vi "Vision Processing.vi"(4 "error in (no error)":errorcluster, 5 "Camera Type":enum16{"206", "1011", "1013"}(ring)=enum."1011") -> ()   [LabVIEW 2012]
uses:
  Robot Global Data.vi
  <vilib>/vision/NI_Vision_Development_Module.lvlib
panel:
  out "Out Cirlcle Info":cluster{dbl, dbl}
  out "Circle Info":cluster{dbl, dbl, dbl}[](array[cluster])
  in  "Range":cluster{"Lower value":sgl, "Upper value":sgl}={"Lower value"=151.52174, "Upper value"=255.0} {"Lower value" scale=0.0..255.0; "Upper value" scale=0.0..255.0}
  out "Out Target Info":cluster{"X":dbl, "Y":dbl, "Distance (ft)":dbl}
  in  "Enable Vision":bool=TRUE
  in  "View":bool
  out "Target Info":T1(array[cluster])
  in  "Area Size Limit %":dbl=0.5
  in  "Particle Count Limit":i32=8
  in  "Score Limits":T2={"Rect Coverage"=60.0, "X Edge Strength"=40.0, "Y Edge Strength"=60.0, "Center"=33.0, "Outer"=50.0}
  in  "View":bool
  out "Processed Image":T3(plugin-control)
  out "Original Image":T3(plugin-control)
  # "Instructions:\nProcessing the reflective tape that is illuminated by a ring light can be based\non color or light intensity.\nParticles within the image are scored by rectangle coverage, aspect ratio, and\nfor being hollow with a bold edge. A particle is considered a target if all scores\nare above the score limits. Particles can be annotated -- surrounded by\na rectangle and scores drawn to the left .\nTo control the number of particles being scored, use the count limit and the size\nlimit."
  # "To debug, Enable using the View button.\nFor color processing, you can click in the image to select the color for processing."
  # "Enable by clicking the View button.\nGreen scores are above the limit, orange are below. Inner/outer rect\nindicates all passed."
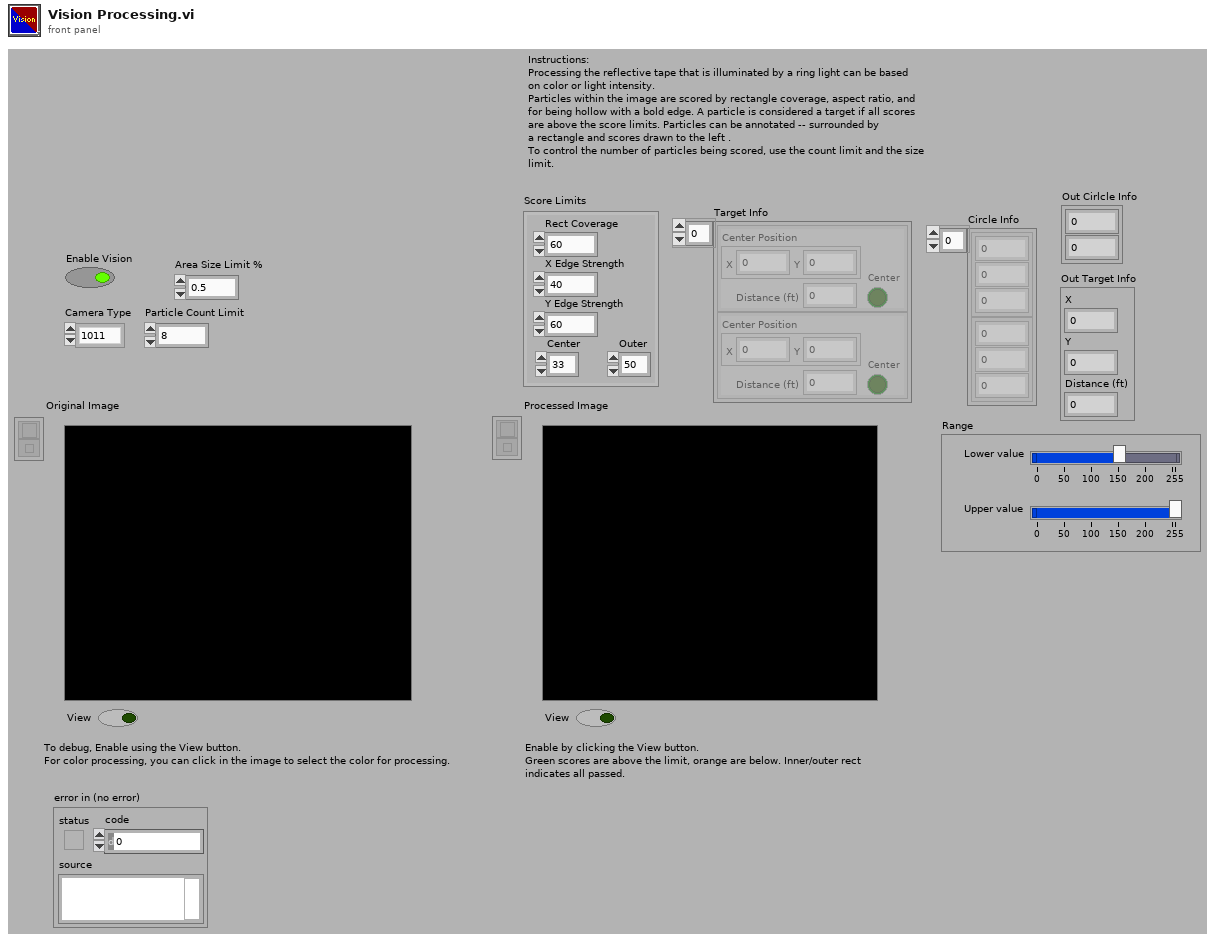
[diagram p1: front panel]
types:
  T1 = cluster{"Center Position":cluster{"X":dbl, "Y":dbl}, "Distance (ft)":dbl, "Center":bool}[]
  T2 = cluster{"Rect Coverage":dbl, "X Edge Strength":dbl, "Y Edge Strength":dbl, "Center":dbl, "Outer":dbl}
  T3 = typedef "IMAQ Image.ctl" = refnum<image>
  T4 = typedef "Image Type" = u32
  T5 = typedef "WPI_CameraDevRef.ctl" = cluster{"Camera Address":string, "CameraStatus":errorcluster, "Acquire Image Notifier":refnum<notifier>}
  T6 = cluster{"Position":cluster{"X":dbl, "Y":dbl}, "Distance (ft)":dbl, "Center":bool}[]
  T7 = typedef "WPI_CameraImageSize.ctl" = enum16{"640x480", "320x240", "160x120"}
  T8 = cluster{cluster{"Left":dbl, "Top":dbl, "Right":dbl, "Bottom":dbl}, "Scores":dbl[], cluster{"Long":dbl, "Short":dbl}}[]
  T9 = cluster{"Target Center (-1 to 1)":cluster{"X":dbl, "Y":dbl}, "Distance (ft)":dbl, "Center Target":bool}
  T10 = cluster{"Target Center (-1 to 1)":cluster{"X":dbl, "Y":dbl}, "Distance (ft)":dbl, "Center Target":bool}[]
  T11 = cluster{"Left":dbl, "Top":dbl, "Right":dbl, "Bottom":dbl}
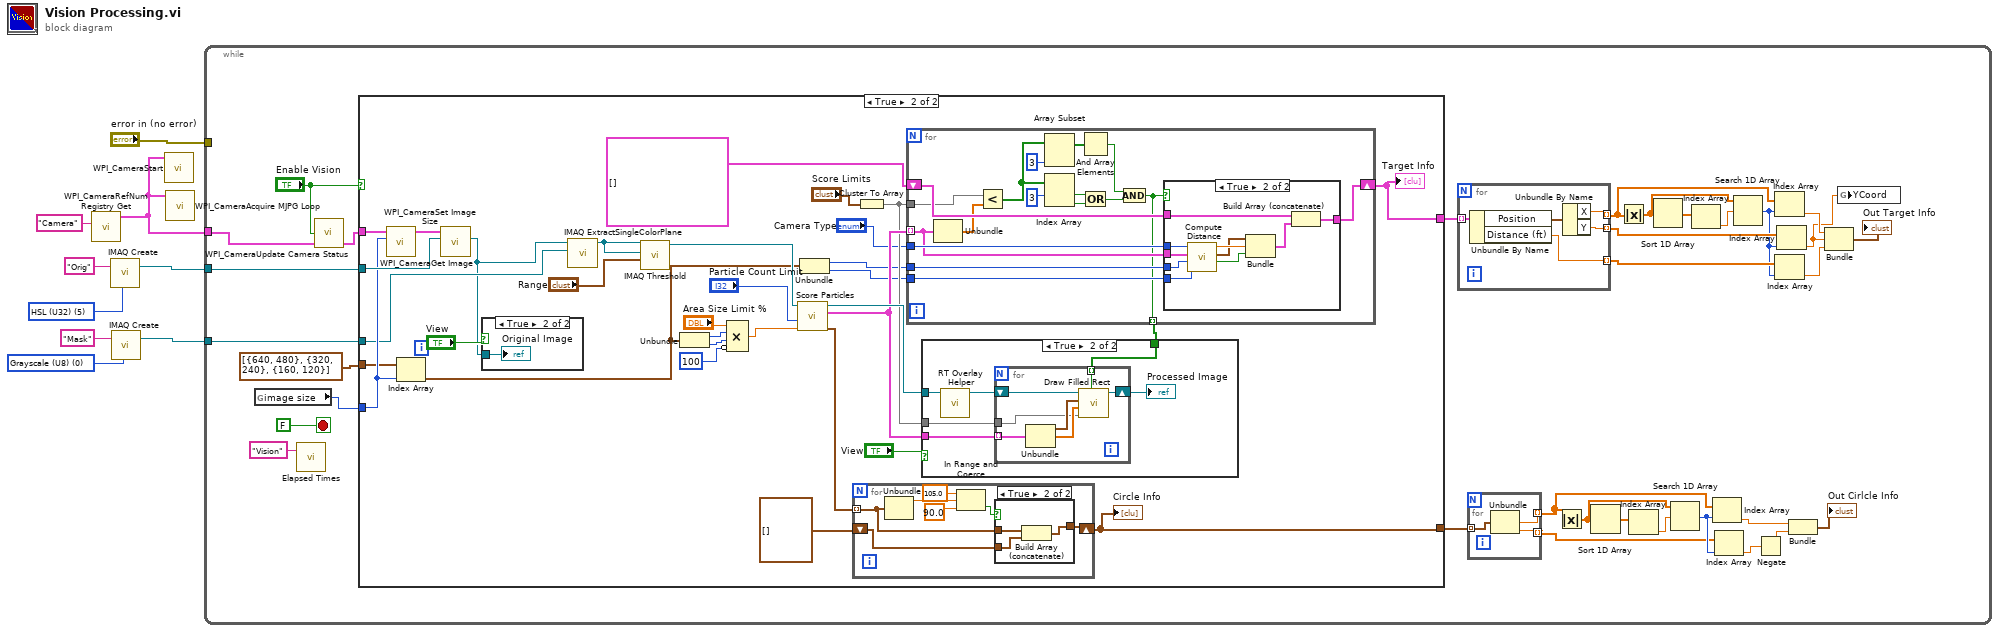
[diagram p0: block diagram]
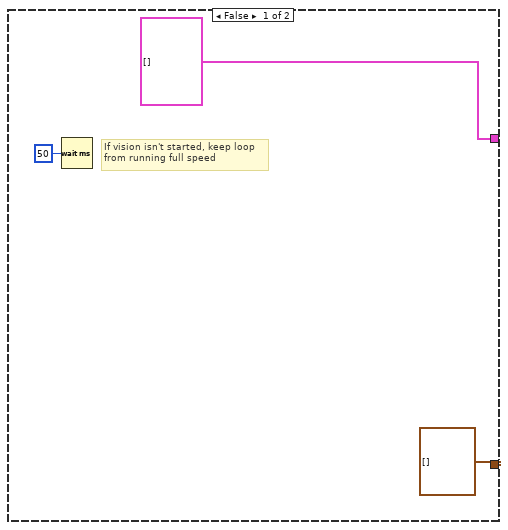
[diagram p2: hidden frame]
diagram:
  w5 = T4 0 items=["Grayscale (U8)", "Grayscale (I16)", "Grayscale (SGL)", "Complex (CSG)", "RGB (U32)", "HSL (U32)", "RGB (U64)", "Grayscale (U16)"] ("Image Type")
  w8 = T4 5 items=["Grayscale (U8)", "Grayscale (I16)", "Grayscale (SGL)", "Complex (CSG)", "RGB (U32)", "HSL (U32)", "RGB (U64)", "Grayscale (U16)"] ("Image Type")
  n1 = call <vilib>:"WPI_CameraRefNum Registry Get.vi"("refnum name"="Camera") -> ("CameraDevRef"=w1:T5)  [unwired: 9 in, 1 out]
  n2 = call "IMAQ Create"("Image Name"="Orig", "Image Type"=w8) -> ("New Image"=w7:T3)  [unwired: 2 in, 2 out]
  n3 = call "IMAQ Create"("Image Name"="Mask", "Image Type"=w5) -> ("New Image"=w3:T3)  [unwired: 2 in, 2 out]
  n4 = call <vilib>:"WPI_CameraStart.vi"("CameraDevRef"=w1) -> ()  [unwired: 9 in, 2 out]
  n5 = call <vilib>:"WPI_CameraAcquire MJPG Loop.vi"("CameraDevRef"=w1) -> ()  [unwired: 11 in]
  n6 = while {
    tunnel: w7 -> [w40]
    tunnel: w1 -> [w39]
    tunnel: "error in (no error)" -> [_]
    tunnel: w3 -> [w37]
    stop <- FALSE stop-if-true
    n7 = global read "Robot Global Data.vi" "image size"() -> (w11:T7)
    n8 = call "Elapsed Times.vi"("Call Name"="Vision") -> ()  [unwired: 2 in, 1 out]
    n9 = call <vilib>:"WPI_CameraUpdate Camera Status.vi"("CameraDevRef In"=w39, "Enable Vision"="Enable Vision") -> ("CameraDevRef Out"=w38:T5)  [unwired: 3 in]
    n10 = case shown="True" "Enable Vision" {
      tunnel: w40 -> [_ w79]
      tunnel: w38 -> [_ w77]
      tunnel: w11 -> [_ w74]
      tunnel: w37 -> [_ w70]
      tunnel: cluster{i32, i32}[] [{640, 480}, {320, 240}, {160, 120}] -> [_ w73]
      tunnel: [T6 [] w64] -> w33
      tunnel: [cluster{dbl, dbl, dbl}[] [] ("Circle Info 2") w54] -> w17
      frame False {
        # "If vision isn't started, keep loop\nfrom running full speed"
        n11 = Wait (ms)(milliseconds to wait=u32 50) -> ()  [unwired: 1 out]
      }
      frame True {
        n12 = call <vilib>:"WPI_CameraSet Image Size.vi"("Image Size"=w74, "CameraDevRef"=w77) -> ("CameraDevRef Out"=w78:T5)  [unwired: 8 in, 1 out]
        n13 = Index Array(array=w73, index=w74) -> (element=w65:cluster{i32, i32})
        n14 = call <vilib>:"WPI_CameraGet Image.vi"("Image"=w79, "CameraDevRef"=w78) -> ("Image Out"=w69:T3)  [unwired: 7 in, 2 out]
        n15 = case shown="True" "View" {
          tunnel: w69 -> [_ w137]
          frame False {
          }
          frame True {
            "Original Image" <- w137
          }
        }
        n16 = call "IMAQ ExtractSingleColorPlane"("Image Dst"=w70, "Image Src"=w69) -> ("Image Dst Out"=w62:T3)  [unwired: 8 in, 1 out]
        n17 = call "IMAQ Threshold"("Range"="Range", "Image Dst"=w62, "Image Src"=w62) -> ("Image Dst Out"=w75:T3)  [unwired: 3 in, 5 out]
        n18 = Unbundle(w65) -> (w59:i32, w58:i32)
        n19 = Compound Arithmetic op=MULTIPLY("Area Size Limit %", w59, w58, invert 100 ("length")) -> (w56:dbl)
        n20 = call "Score Particles.vi"("Area Size Limit"=w56, "Particle Count Limit"="Particle Count Limit", "Image Refnum in"=w75) -> ("Circle Info"=w55:cluster{dbl, dbl, dbl}[], "Scored Particle Info"=w82:T8, "Image Refnum out"=w84:T3)  [unwired: 6 in]
        n21 = Unbundle(w65) -> (w72:i32, w71:i32)
        n22 = for {
          tunnel: w55 -> [w87] mode=indexing
          shift-right: [w85] -> w54
          shift-left: cluster{dbl, dbl, dbl}[] [] ("Circle Info") -> [w86]
          n23 = Unbundle(w87) -> (w91:dbl)  [unwired: 2 out]
          n24 = In Range and Coerce(upper limit=105.0, x=w91, lower limit=90.0) -> (In Range?=w88:bool)  [unwired: 1 out]
          n25 = case shown="True" w88 {
            tunnel: w87 -> [_ w95]
            tunnel: w86 -> [w92 w94]
            tunnel: [w92 w93] -> w85
            frame False {
            }
            frame True {
              n26 = Build Array (concatenate)(w95, w94) -> (w93:cluster{dbl, dbl, dbl}[])
            }
          }
        }
        "Circle Info" <- w54
        n27 = Cluster To Array(cluster="Score Limits") -> (array=w80:dbl[])
        n28 = for {
          shift-right: [w111] -> w64
          shift-left: T6 [] -> [w112]
          tunnel: w72 -> [w110]
          tunnel: w82 -> [w105] mode=indexing
          tunnel: w80 -> [w107]
          tunnel: "Camera Type" -> [w109]
          tunnel: w71 -> [w106]
          tunnel: [w96] -> w66 mode=indexing
          n29 = Unbundle(w105) -> ("Scores"=w108:dbl[])  [unwired: 2 out]
          n30 = Less?(x=w107, y=w108) -> (x < y?=w97:bool[])
          n31 = Array Subset(array=w97, length=3) -> (w99:bool[])  [unwired: 1 in]
          n32 = Index Array(array=w97, index #1=3 ("length")) -> (element #1=w101:bool, element #2=w102:bool)  [unwired: 1 in]
          n33 = And Array Elements(Boolean array=w99) -> (logical AND=w104:bool)
          n34 = Or(x=w101, y=w102) -> (x .or. y?=w103:bool)
          n35 = And(x=w104, y=w103) -> (x .and. y?=w96:bool)
          n36 = case shown="True" w96 {
            tunnel: w112 -> [w113 w123]
            tunnel: [w113 w122] -> w111
            tunnel: w110 -> [_ w120]
            tunnel: w109 -> [_ w119]
            tunnel: w106 -> [_ w118]
            tunnel: w105 -> [_ w117]
            frame False {
            }
            frame True {
              n37 = call "Compute Distance.vi"("Y Image Resolution"=w118, "X Image Resolution"=w120, "Particle Scores"=w117, "Camera Type"=w119) -> ("Center Target"=w114:bool, "Target Center (-1 to 1)"=w115:cluster{"X":dbl, "Y":dbl}, "Distance (ft)"=w116:dbl)  [unwired: 5 in]
              n38 = Bundle("Target Center (-1 to 1)"=w115, "Distance (ft)"=w116, "Center Target"=w114) -> (w121:T9)  [unwired: 1 in]
              n39 = Build Array (concatenate)(w123, w121) -> (w122:T10)
            }
          }
        }
        "Target Info" <- w64
        n40 = case shown="True" "View" {
          tunnel: w84 -> [_ w126]
          tunnel: w82 -> [_ w128]
          tunnel: w80 -> [_ w127]
          tunnel: w66 -> [_ w124]
          frame False {
          }
          frame True {
            n41 = call "RT Overlay Helper.vi"("Refnum in"=w126) -> ("Refnum out"=w129:T3)  [unwired: 10 in]
            n42 = for {
              shift-right: [w135] -> w125
              shift-left: w129 -> [w136]
              tunnel: w128 -> [w132] mode=indexing
              tunnel: w127 -> [w131]
              tunnel: w124 -> [w130] mode=indexing
              n43 = Unbundle(w132) -> (w133:T11, "Scores"=w134:dbl[])  [unwired: 1 out]
              n44 = call "Draw Filled Rect.vi"("Limit Passed"=w130, "Limits"=w131, "Scores"=w134, "Bounding Box"=w133, "image in"=w136) -> ("image out"=w135:T3)  [unwired: 6 in]
            }
            "Processed Image" <- w125
          }
        }
      }
    }
    n45 = for {
      tunnel: w33 -> [w49] mode=indexing
      tunnel: [w47] -> w29 mode=indexing
      tunnel: [w46] -> w28 mode=indexing
      tunnel: [w45] -> w27 mode=indexing
      n46 = Unbundle By Name(w49) -> ("Position"=w48:cluster{"X":dbl, "Y":dbl}, "Distance (ft)"=w45:dbl)
      n47 = Unbundle By Name(w48) -> ("X"=w47:dbl, "Y"=w46:dbl)
    }
    n48 = for {
      tunnel: w17 -> [w44] mode=indexing
      tunnel: [w42] -> w21 mode=indexing
      tunnel: [w43] -> w22 mode=indexing
      n49 = Unbundle(w44) -> (w42:dbl, w43:dbl)  [unwired: 1 out]
    }
    n50 = Absolute Value(x=w21) -> (abs(x)=w19:dbl[])
    n51 = Sort 1D Array(array=w19) -> (sorted array=w18:dbl[])
    n52 = Absolute Value(x=w29) -> (abs(x)=w31:dbl[])
    n53 = Index Array(array=w18) -> (element=w20:dbl)  [unwired: 1 in]
    n54 = Sort 1D Array(array=w31) -> (sorted array=w32:dbl[])
    n55 = Search 1D Array(1D array=w19, element=w20) -> (index of element=w23:i32)  [unwired: 1 in]
    n56 = Index Array(array=w32) -> (element=w30:dbl)  [unwired: 1 in]
    n57 = Index Array(array=w21, index=w23) -> (element=w16:dbl)
    n58 = Index Array(array=w22, index=w23) -> (element=w15:dbl)
    n59 = Search 1D Array(1D array=w31, element=w30) -> (index of element=w26:i32)  [unwired: 1 in]
    n60 = Negate(x=w15) -> (-x=w14:dbl)
    n61 = Index Array(array=w29, index=w26) -> (element=w25:dbl)
    n62 = Index Array(array=w27, index=w26) -> (element=w24:dbl)
    n63 = Index Array(array=w28, index=w26) -> (element=w10:dbl)
    n64 = Bundle(w16, w14) -> (→"Out Cirlcle Info":cluster{dbl, dbl})  [unwired: 1 in]
    n65 = Bundle("X"=w25, "Y"=w10, "Distance (ft)"=w24) -> (→"Out Target Info":cluster{"X":dbl, "Y":dbl, "Distance (ft)":dbl})  [unwired: 1 in]
    n66 = global write "Robot Global Data.vi" "YCoord"(w10) -> ()
  }
